vi "Day 5.1 - overlap.vi"(11 "input":string[](array[string])) -> (3 "output":u32)   [LabVIEW 2021]
uses:
  Controls/Thermal position.ctl
  Controls/vent position.ctl
panel:
  out "Intensity Graph":i32[][](graph)
  out "vents":i32[][](array[numeric])
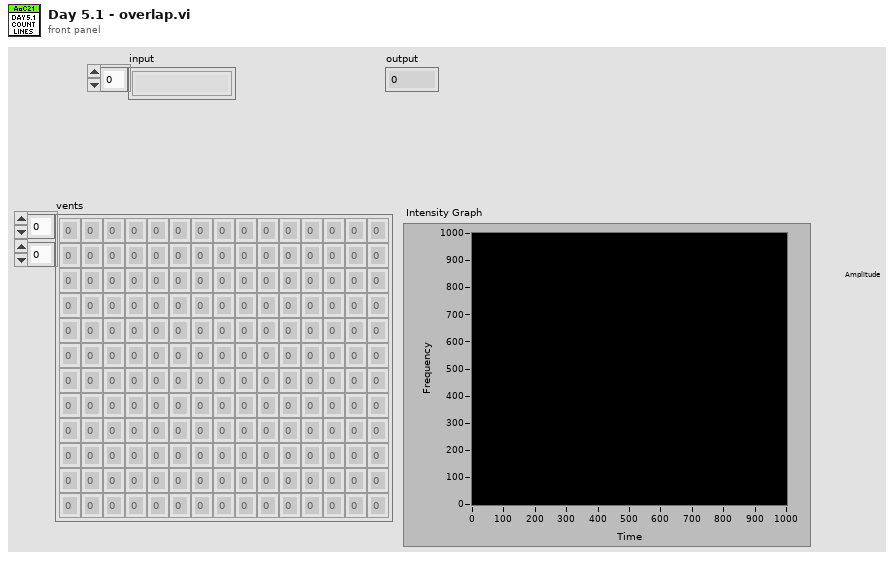
[diagram p1: front panel]
types:
  T1 = typedef "Thermal position.ctl" = cluster{"Start Vent position":T2, "End Vent position":T2}
  T2 = typedef "vent position.ctl" = cluster{"x":i32, "y":i32}
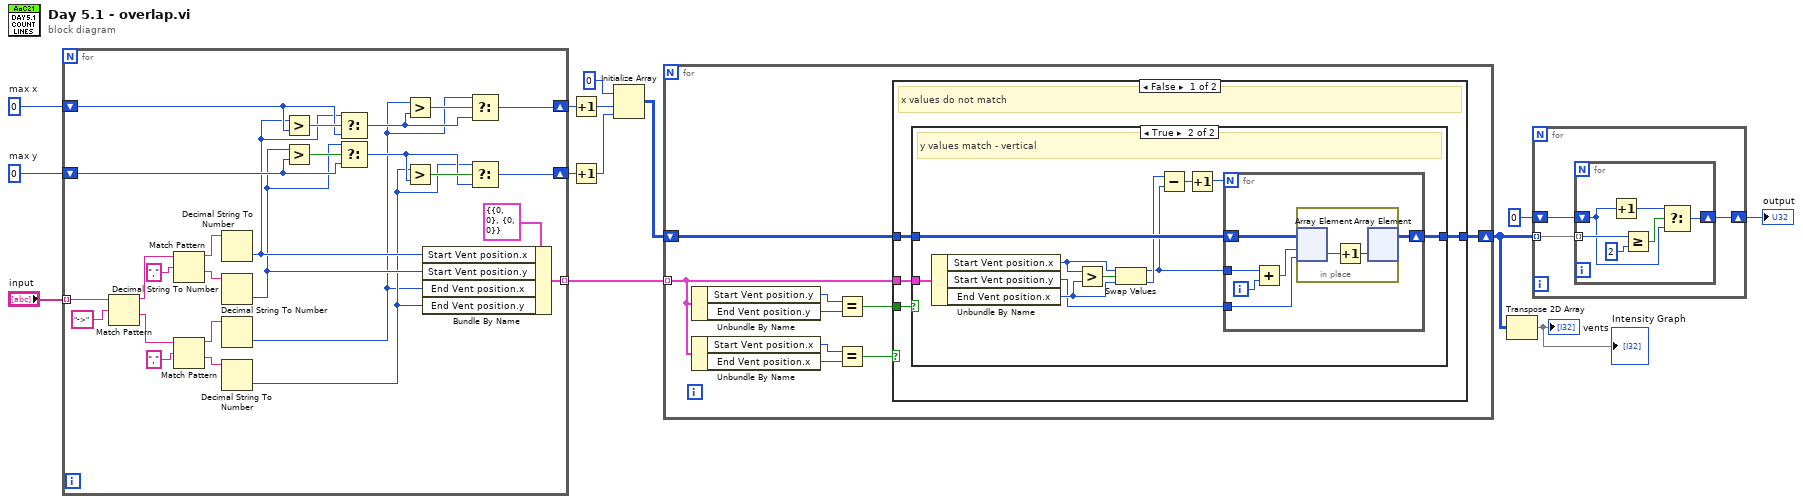
[diagram p0: block diagram]
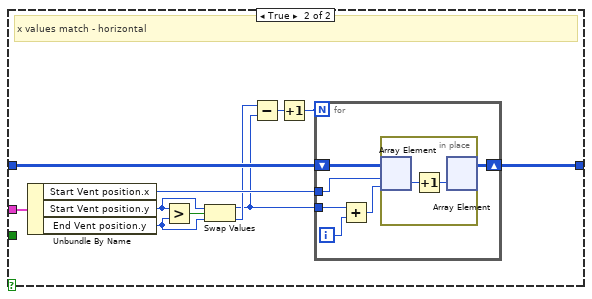
[diagram p3: hidden frame]
diagram:
  w11 = 0  # max y
  w12 = 0  # max x
  n1 = for {
    tunnel: "input" -> [w40] mode=indexing
    tunnel: [w29] -> w13 mode=indexing
    shift-right: [w25] -> w10
    shift-left: w12 -> [w27]
    shift-right: [w20] -> w9
    shift-left: w11 -> [w19]
    n2 = Match Pattern(string=w40, regular expression="->") -> (before substring=w38:string, after substring=w35:string)  [unwired: 1 in, 2 out]
    n3 = Match Pattern(string=w38, regular expression=",") -> (before substring=w32:string, after substring=w31:string)  [unwired: 1 in, 2 out]
    n4 = Match Pattern(string=w35, regular expression=",") -> (before substring=w34:string, after substring=w33:string)  [unwired: 1 in, 2 out]
    n5 = Decimal String To Number(string=w32) -> (number=w18:i32)  [unwired: 2 in, 1 out]
    n6 = Decimal String To Number(string=w31) -> (number=w17:i32)  [unwired: 2 in, 1 out]
    n7 = Decimal String To Number(string=w34) -> (number=w15:i32)  [unwired: 2 in, 1 out]
    n8 = Decimal String To Number(string=w33) -> (number=w16:i32)  [unwired: 2 in, 1 out]
    n9 = Greater?(x=w18, y=w27) -> (0:w28:bool)
    n10 = Greater?(x=w17, y=w19) -> (0:w23:bool)
    n11 = Select(t=w18, s=w28, f=w27) -> (s? t:f=w24:i32)
    n12 = Select(t=w17, s=w23, f=w19) -> (s? t:f=w21:i32)
    n13 = Greater?(x=w15, y=w24) -> (0:w26:bool)
    n14 = Greater?(x=w16, y=w21) -> (0:w22:bool)
    n15 = Bundle By Name(cluster=T1 {"Start Vent position"={"x"=0, "y"=0}, "End Vent position"={"x"=0, "y"=0}} ("Hydrothermal"), "Start Vent position.x"=w18, "Start Vent position.y"=w17, "End Vent position.x"=w15, "End Vent position.y"=w16) -> (w29:T1)
    n16 = Select(t=w15, s=w26, f=w24) -> (s? t:f=w25:i32)
    n17 = Select(t=w16, s=w22, f=w21) -> (s? t:f=w20:i32)
  }
  n18 = Increment(x=w10) -> (x+1=w7:i32)
  n19 = Increment(x=w9) -> (x+1=w3:i32)
  n20 = Initialize Array(0, w7, w3) -> (w8:i32[][])
  n21 = for {
    tunnel: w13 -> [w42] mode=indexing
    shift-right: [w41] -> w4
    shift-left: w8 -> [w44]
    n22 = Unbundle By Name(w42) -> ("Start Vent position.y"=w49:i32, "End Vent position.y"=w48:i32)
    n23 = Unbundle By Name(w42) -> ("Start Vent position.x"=w46:i32, "End Vent position.x"=w45:i32)
    n24 = Equal?(x=w49, y=w48) -> (x = y?=w43:bool)
    n25 = Equal?(x=w46, y=w45) -> (x = y?=w47:bool)
    n26 = case shown="False" w47 {
      tunnel: w44 -> [w51 w84]
      tunnel: [w50 w77] -> w41
      tunnel: w43 -> [w53 _]
      tunnel: w42 -> [w52 w74]
      frame False {
        # "x values do not match"
        n27 = case shown="True" w53 {
          tunnel: [w54 w62] -> w50
          tunnel: w52 -> [_ w65]
          tunnel: w51 -> [w54 w61]
          frame False {
            # "y values do not match"
          }
          frame True {
            # "y values match - vertical"
            n28 = Unbundle By Name(w65) -> ("Start Vent position.x"=w58:i32, "Start Vent position.y"=w56:i32, "End Vent position.x"=w57:i32)
            n29 = Greater?(x=w58, y=w57) -> (0:w64:bool)
            n30 = Swap Values(12:w58, 13:w64, 14:w57) -> (1:w59:i32, 3:w60:i32)
            n31 = Subtract(x=w60, y=w59) -> (x-y=w63:i32)
            n32 = Increment(x=w63) -> (x+1=w55:i32)
            n33 = for {
              N: w55 -> [_]
              tunnel: w56 -> [w67]
              tunnel: w59 -> [w70]
              shift-right: [w66] -> w62
              shift-left: w61 -> [w69]
              i -> [w71]
              n34 = Add(x=w70, y=w71) -> (x+y=w68:i32)
              n35 = in-place {
                n36 = in-place-array #1(w69, w68, w67) -> (w73:i32)
                n37 = Increment(x=w73) -> (x+1=w72:i32)
                n38 = in-place-array #1(w72) -> (w66:i32[][])  [unwired: 2 out]
              }
            }
          }
        }
      }
      frame True {
        # "x values match - horizontal"
        n39 = Unbundle By Name(w74) -> ("Start Vent position.x"=w83:i32, "Start Vent position.y"=w81:i32, "End Vent position.y"=w80:i32)
        n40 = Greater?(x=w81, y=w80) -> (0:w82:bool)
        n41 = Swap Values(12:w81, 13:w82, 14:w80) -> (1:w75:i32, 3:w78:i32)
        n42 = Subtract(x=w78, y=w75) -> (x-y=w79:i32)
        n43 = Increment(x=w79) -> (x+1=w76:i32)
        n44 = for {
          N: w76 -> [_]
          tunnel: w83 -> [w89]
          tunnel: w75 -> [w87]
          shift-right: [w85] -> w77
          shift-left: w84 -> [w90]
          i -> [w88]
          n45 = Add(x=w87, y=w88) -> (x+y=w86:i32)
          n46 = in-place {
            n47 = in-place-array #2(w90, w89, w86) -> (w92:i32)
            n48 = Increment(x=w92) -> (x+1=w91:i32)
            n49 = in-place-array #2(w91) -> (w85:i32[][])  [unwired: 2 out]
          }
        }
      }
    }
  }
  n50 = Transpose 2D Array(2D array=w4) -> (transposed array=→"vents" →"Intensity Graph":i32[][])
  n51 = for {
    tunnel: w4 -> [w95] mode=indexing
    shift-right: [w93] -> w5
    shift-left: 0 -> [w94]
    n52 = for {
      tunnel: w95 -> [w101] mode=indexing
      shift-right: [w96] -> w93
      shift-left: w94 -> [w98]
      n53 = Increment(x=w98) -> (x+1=w97:i32)
      n54 = Greater Or Equal?(x=w101, y=2) -> (x >= y?=w99:bool)
      n55 = Select(t=w97, s=w99, f=w98) -> (s? t:f=w96:i32)
    }
  }
  "output" <- w5
